vi "OnDataChange.vi"(0 "Controller Template in":refnum<class "DisplayerUI.lvclass">, 1 "DataExchange":T1, 3 "error in (no error)":errorcluster) -> (7 "Controller Template out":refnum<class "DisplayerUI.lvclass">, 10 "error out":errorcluster)   [LabVIEW 2020, in "Displayer.lvlib" / "DisplayerUI.lvlib" / "DisplayerUI.lvclass"]
uses:
  DisplayerUI.lvclass
  Model/Hardware Abstraction Layer/Component/Device/Device/DataExchange.ctl
  Interface/DataListener/DataListener.lvclass
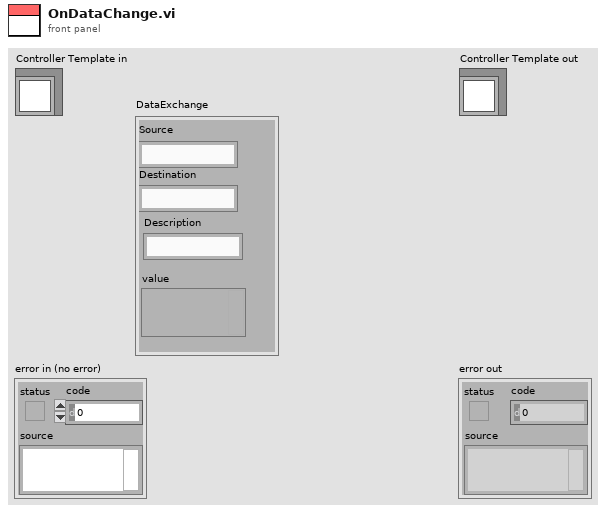
[diagram p1: front panel]
types:
  T1 = typedef "DataListener.lvclass/DataExchange.ctl" = cluster{"Source":string, "Destination":string, "Description":string, "value":variant}
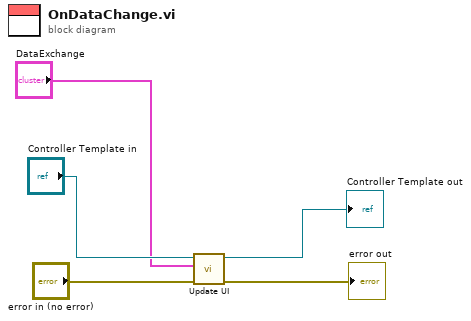
[diagram p0: block diagram]
diagram:
  n1 = call-dynamic "Update UI.vi"("error in (no error)"="error in (no error)", "DataExchange"="DataExchange", "Controller Template in"="Controller Template in") -> ("error out"=→"error out":errorcluster, "Controller Template out"=→"Controller Template out":refnum<class "DisplayerUI.lvclass">)  [unwired: 7 in]
